vi "(SubVI)Update Log.vi"(7 "Log Ref":refnum<vi>, 8 "error in (no error)":errorcluster caption="에러 입력(에러 없음)", 11 "Log":string) -> (0 "error out":errorcluster caption="에러 출력", 3 "Log out":string)   [LabVIEW 2020]
panel:
  # "(SubVI)Update Log.vi By hspark\n\nDescription : Log 문자열 인디케이터에 Log를 추가하는 VI\n\nInput : \n1. Log : Log 내용\n2. Log Ref : Log를 남길 문자열 인디케이터 참조. 입력하지 않은 경우 Log를 남기지 않음\n\nOutput : \n1. Log out : Log 내용 출력\n\nLabVIEW Version : 2020 SP1 이상\n\nNote : \nLog 인디케이터의 최대 라인 수를 2000으로 제한함. \n문자열 컨트롤/인디케이터의 내용이 길어지면 PC 성능이 떨어질 수 있음.\n최대 라인이 2000줄 이상 필요한 경우 상수 값 수정하되 버벅이지 않는지 테스트 필요.\n\nUpdate : 2021.10.06"
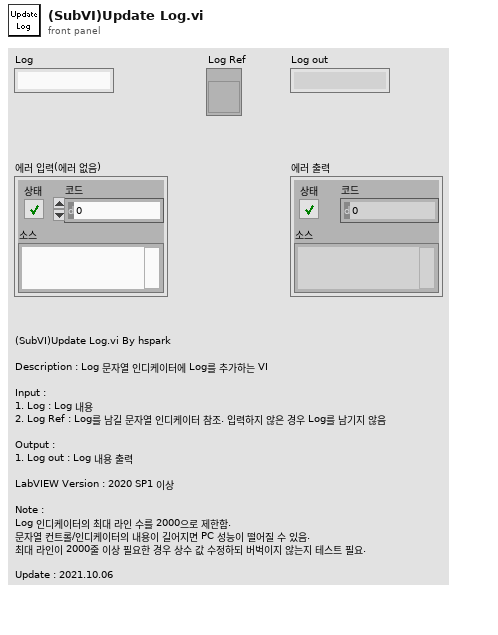
[diagram p1: front panel]
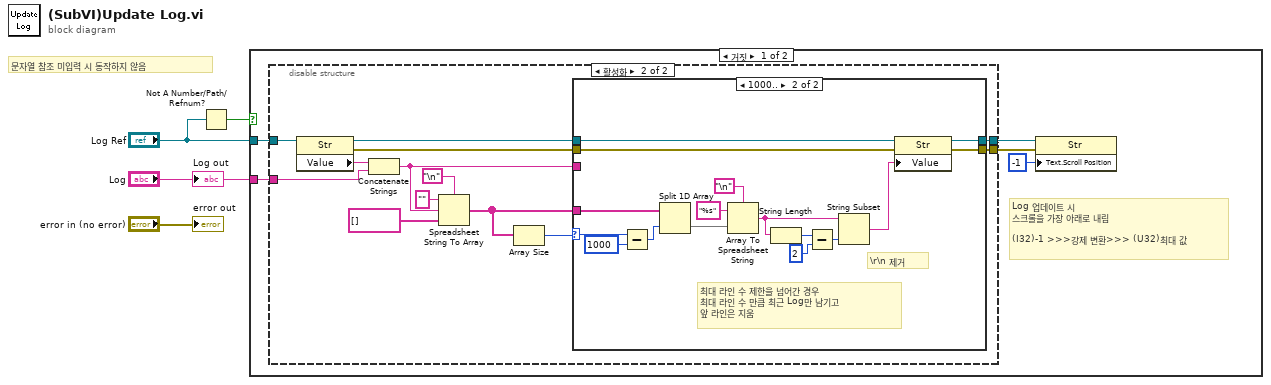
[diagram p0: block diagram]
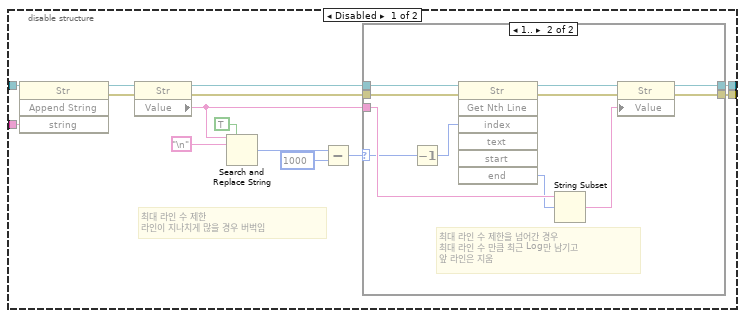
[diagram p2: hidden frame]
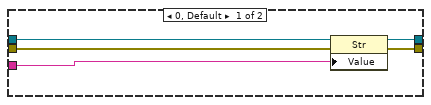
[diagram p4: hidden frame]
diagram:
  # "문자열 참조 미입력 시 동작하지 않음"
  n1 = Not A Number/Path/Refnum?(number/path/refnum="Log Ref") -> (NaN/Path/Refnum?=w1:bool)
  n2 = case shown="거짓" w1 {
    tunnel: "Log" -> [w9 _]
    tunnel: "Log Ref" -> [w7 _]
    frame False {
      # "Log 업데이트 시\n스크롤을 가장 아래로 내림\n\n(I32)-1 >>>강제 변환>>> (U32)최대 값"
      n3 = disable-structure shown="활성화" {
        disable-tunnel: w9 -> [w23 w47]
        disable-tunnel: w7 -> [w21 w49]
        disable-tunnel: [w15 w38] -> w6
        disable-tunnel: [w14 w37] -> w5
        frame Disabled {
          # "최대 라인 수 제한\n라인이 지나치게 많을 경우 버벅임"
          n4 = invoke class="Str" method="Append String"(reference=w21, "string"=w23) -> (reference out=w20:refnum<vi>, error out=w22:errorcluster)  [unwired: 2 in, 2 out]
          n5 = property class="Str"(reference=w20, error in=w22) -> (reference out=w17:refnum<vi>, error out=w16:errorcluster, "Value"=w13:string)
          n6 = Search and Replace String(replace all?=TRUE ("모두 대체? (거짓)"), input string=w13, search string="\n") -> (number of replacements=w12:i32)  [unwired: 5 in, 3 out]
          n7 = Subtract(x=w12, y=1000 ("x")) -> (x-y=w10:i32)
          n8 = case shown="1.." w10 {
            selector: w10 -> [_ w27]
            tunnel: w17 -> [w25 w34]
            tunnel: w16 -> [w24 w36]
            tunnel: [w25 w31] -> w15
            tunnel: [w24 w33] -> w14
            tunnel: w13 -> [_ w30]
            frame ..0 {
            }
            frame 1.. {
              # "최대 라인 수 제한을 넘어간 경우\n최대 라인 수 만큼 최근 Log만 남기고\n앞 라인은 지움"
              n9 = Decrement(x=w27) -> (x-1=w26:i32)
              n10 = invoke class="Str" method="Get Nth Line"(reference=w34, error in=w36, "index"=w26) -> (reference out=w32:refnum<vi>, error out=w35:errorcluster, "end"=w29:u32)  [unwired: 4 in, 4 out]
              n11 = String Subset(string=w30, offset (0)=w29) -> (substring=w28:string)  [unwired: 1 in]
              n12 = property class="Str"(reference=w32, error in=w35, "Value"=w28) -> (reference out=w31:refnum<vi>, error out=w33:errorcluster)
            }
          }
        }
        frame Enabled {
          n13 = property class="Str"(reference=w49) -> (reference out=w46:refnum<vi>, error out=w41:errorcluster, "Value"=w48:string)  [unwired: 1 in]
          n14 = Concatenate Strings(w48, w47) -> (w39:string)
          n15 = Spreadsheet String To Array(delimiter (Tab)="\n", format string="" ("포맷 문자열"), spreadsheet string=w39, array type (2D Dbl)=string[] []) -> (array=w40:string[])
          n16 = Array Size(array=w40) -> (size(s)=w42:i32)
          n17 = case shown="1000.." w42 {
            selector: w42 -> [_ w65]
            tunnel: w46 -> [w54 w68]
            tunnel: [w52 w69] -> w38
            tunnel: [w51 w70] -> w37
            tunnel: w41 -> [w53 w67]
            tunnel: w40 -> [_ w66]
            tunnel: w39 -> [w50 _]
            frame 0, Default {
              n18 = property class="Str"(reference=w54, error in=w53, "Value"=w50) -> (reference out=w52:refnum<vi>, error out=w51:errorcluster)
            }
            frame 1000.. {
              # "\\r\\n 제거"
              # "최대 라인 수 제한을 넘어간 경우\n최대 라인 수 만큼 최근 Log만 남기고\n앞 라인은 지움"
              n19 = Subtract(x=w65, y=1000) -> (x-y=w63:i32)
              n20 = Split 1D Array(array=w66, index=w63) -> (second subarray=w62:string[])  [unwired: 1 out]
              n21 = Array To Spreadsheet String(delimiter (Tab)="\n", array=w62, 3:"%s" ("포맷 문자열")) -> (spreadsheet string=w57:string)
              n22 = String Length(string=w57) -> (length=w59:i32)
              n23 = Subtract(x=w59, y=2) -> (x-y=w58:i32)
              n24 = String Subset(string=w57, length (rest)=w58) -> (substring=w56:string)  [unwired: 1 in]
              n25 = property class="Str"(reference=w68, error in=w67, "Value"=w56) -> (reference out=w69:refnum<vi>, error out=w70:errorcluster)
            }
          }
        }
      }
      n26 = property class="Str"(reference=w6, error in=w5, "Text.Scroll Position"=-1 ("텍스트.스크롤 위치")) -> ()  [unwired: 2 out]
    }
    frame True {
    }
  }
  "error out" <- "error in (no error)"
  "Log out" <- "Log"
